vi "Retrieve Logic and Convert DI.vi"(7 "bypass (F)":bool, 8 "error in (no error)":errorcluster, 9 "RawValue in":bool, 10 "IOName":string, 11 "DAQ Node Dict DVR":T1) -> (0 "error out":errorcluster, 1 "ConvertedValue Out":bool, 2 "IOName out":string, 3 "DAQ Node Dict DVR out":T1)   [LabVIEW 2017, in "DAQ.lvclass"]
doc: "Developed by Kevin Thompson\nkevin@thompsonengineering.net\n\nCopyright 2018-2020\nThompson Engineering, LLC"
uses:
  DAQ.lvclass
  <vilib>/TELLC/Dynamic CVT API/TD Dynamic CVT DVR--ref.ctl
  DataTypes/TD DI Channel--cluster.ctl
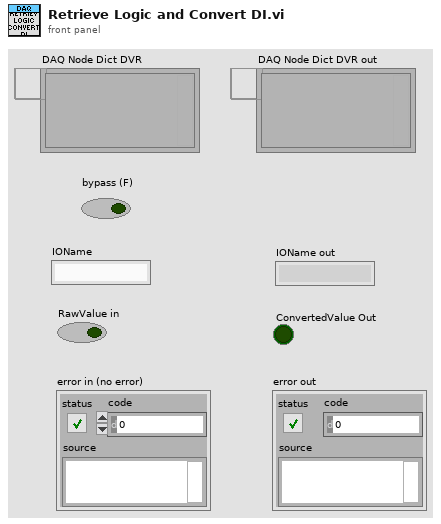
[diagram p1: front panel]
types:
  T1 = typedef "TD Dynamic CVT DVR--ref.ctl" = refnum<data-value>
  T2 = typedef "DAQ.lvclass/TD DI Channel--cluster.ctl" = cluster{"DevName":string, "IOName":string, "IOPath":string, "SchemName":string, "logic":enum16{"Lo", "Hi"}, "Index":i32}
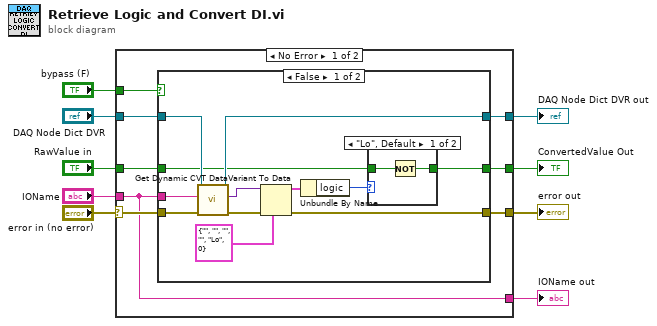
[diagram p0: block diagram]
diagram:
  n1 = case shown="No Error" "error in (no error)" {
    selector: "error in (no error)" -> [w12 w38]
    tunnel: [w17 w37] -> w9
    tunnel: [w16 w38] -> w8
    tunnel: "IOName" -> [w10 w36]
    tunnel: "DAQ Node Dict DVR" -> [w15 w39]
    tunnel: [w14 w39] -> w5
    tunnel: "RawValue in" -> [w13 w37]
    tunnel: "bypass (F)" -> [w11 _]
    tunnel: [w10 w36] -> w1
    frame No Error {
      n2 = case shown="False" w11 {
        tunnel: [w19 w34] -> w17
        tunnel: [w22 w33] -> w16
        tunnel: w10 -> [w26 _]
        tunnel: w15 -> [w25 w35]
        tunnel: [w24 w35] -> w14
        tunnel: w13 -> [w20 w34]
        tunnel: w12 -> [w23 w33]
        frame False {
          n3 = call <vilib>:"Get Dynamic CVT Data.vi"("error in (no error)"=w23, "DataName"=w26, "dCVT DVR"=w25) -> ("error out"=w28:errorcluster, "value"=w27:variant, "dCVT DVR out"=w24:T1)  [unwired: 5 in, 1 out]
          n4 = Variant To Data(error in=w28, type=T2 {"DevName"="", "IOName"="", "IOPath"="", "SchemName"="", "logic"=enum."Lo", "Index"=0} ("DI"), Variant=w27) -> (data=w29:T2, error out=w22:errorcluster)
          n5 = Unbundle By Name(w29) -> ("logic"=w21:enum16{"Lo", "Hi"})
          n6 = case shown="\"Lo\", Default" w21 {
            tunnel: w20 -> [w31 w32]
            tunnel: [w30 w32] -> w19
            frame "Lo", Default {
              n7 = Not(x=w31) -> (.not. x?=w30:bool)
            }
            frame "Hi" {
            }
          }
        }
        frame True {
        }
      }
    }
    frame Error {
    }
  }
  "ConvertedValue Out" <- w9
  "error out" <- w8
  "DAQ Node Dict DVR out" <- w5
  "IOName out" <- w1
